vi "Verify Blink HE.vi"(0 "GEA2 Reference In":refnum<k24>, 1 "SSD":string, 2 "Blinking LED":T1, 5 "Initial Timeout (s)":dbl, 7 "Retry Count":i32, 9 "Max Blink Rate (sec)":dbl, 11 "Error In":errorcluster, 13 "Ignore Brightness?":bool) -> (4 "GEA2 Reference Out":refnum<k24>, 6 "Pass/Fail?":bool, 8 "Report Text":string, 10 "Blink Times (s)":dbl[](array[numeric]), 15 "Error Out":errorcluster)   [LabVIEW 2016, in "TLMB.lvlib"]
doc: "This VI is used to verify that a particular LED is blinking on the HEUI."
uses:
  Projects/TLMB.lvlib
  Q:/Common/DLLs/GEA3/GeaCommunication.dll
  Common/DLLs/GEA3/GeaCommunication.dll
  controls/HEUI_Display_Blink.ctl
  Common/LabVIEW GEA2 Toolkit/LabVIEW_GEA2_Toolkit.lvlibp/type defs/Source_Destination.ctl
  Common/LabVIEW GEA2 Toolkit/LabVIEW_GEA2_Toolkit.lvlibp
panel:
  in  "Standalone":bool
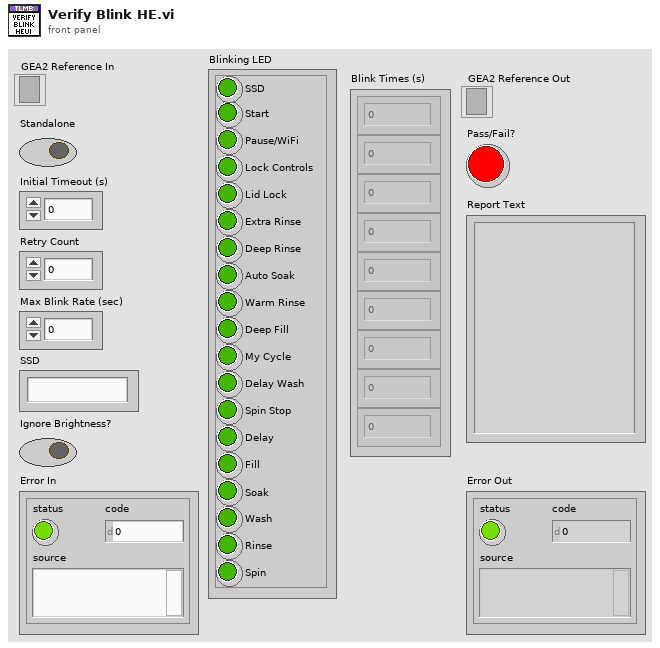
[diagram p1: front panel]
types:
  T1 = typedef "TLMB.lvlib/HEUI_Display_Blink.ctl" = cluster{"Start":bool, "Pause/WiFi":bool, "Lock Controls":bool, "Lid Lock":bool, "Extra Rinse":bool, "Deep Rinse":bool, "Auto Soak":bool, "Warm Rinse":bool, "Deep Fill":bool, "My Cycle":bool, "Delay Wash":bool, "Spin Stop":bool, "Delay":bool, "Fill":bool, "Soak":bool, "Wash":bool, "Rinse":bool, "Spin":bool, "SSD":bool}
  T2 = typedef "LabVIEW_GEA2_Toolkit.lvlibp/Source_Destination.ctl" = cluster{"Source":u8, "Destination":u8}
  T3 = typedef "TLMB.lvlib/HEUI_Display_Care.ctl" = cluster{"SSD":bool, "Cycle Selection":bool, "Stain Selection":bool, "Temp Level":bool, "Soil Level":bool, "Spin Level":bool, "750 Status":bool, "Start":bool, "Pause/WiFi":bool, "Lock Controls":bool, "Lid Lock":bool, "Extra Rinse":bool, "Deep Rinse":bool, "Auto Soak":bool, "Warm Rinse":bool, "Deep Fill":bool, "My Cycle":bool, "Delay Wash":bool, "Spin Stop":bool, "Delay":bool, "Fill":bool, "Soak":bool, "Wash":bool, "Rinse":bool, "Spin":bool}
  T4 = typedef "TLMB.lvlib/HEUI_Display.ctl" = cluster{"SSD":string, "Cycle Selection":T5, "Stain Selection":T6, "Temp Level":T7, "Soil Level":T8, "Spin Level":T9, "750 Status":T10, "Start":bool, "Pause/WiFi":bool, "Lock Controls":bool, "Lid Lock":bool, "Extra Rinse":bool, "Deep Rinse":bool, "Auto Soak":bool, "Warm Rinse":bool, "Deep Fill":bool, "My Cycle":bool, "Delay Wash":bool, "Spin Stop":bool, "Delay":bool, "Fill":bool, "Soak":bool, "Wash":bool, "Rinse":bool, "Spin":bool}
  T5 = typedef "TLMB.lvlib/Cycle Selection Enum.ctl" = enum16{"Colors", "Easy Care", "Delicates", "Hand Wash", "Active Wear", "Speed Wash", "Rinse and Spin", "Drain and Spin", "Basket Clean", "Jeans", "Heavy Duty", "Bulky Items", "Towels", "Whites", "Off", "*Incorrect*"}
  T6 = typedef "TLMB.lvlib/Stain Enum.ctl" = enum16{"Tomato", "Wine", "Blood", "Grass", "Dirt", "Off", "*Incorrect*"}
  T7 = typedef "TLMB.lvlib/Temp Enum.ctl" = enum16{"Hot", "Warm", "Colors", "Cool", "Cold", "Tap Cold", "Off", "*Incorrect*"}
  T8 = typedef "TLMB.lvlib/Soil Enum.ctl" = enum16{"Extra Heavy", "Heavy", "Normal", "Light", "Off", "*Incorrect*"}
  T9 = typedef "TLMB.lvlib/Spin Enum.ctl" = enum16{"Max Spin", "More Spin", "Normal Spin", "No Spin", "Off", "*Incorrect*"}
  T10 = typedef "TLMB.lvlib/750 Status Enum.ctl" = enum16{"Fill", "Wash", "Rinse", "Spin", "Off", "*Incorrect*"}
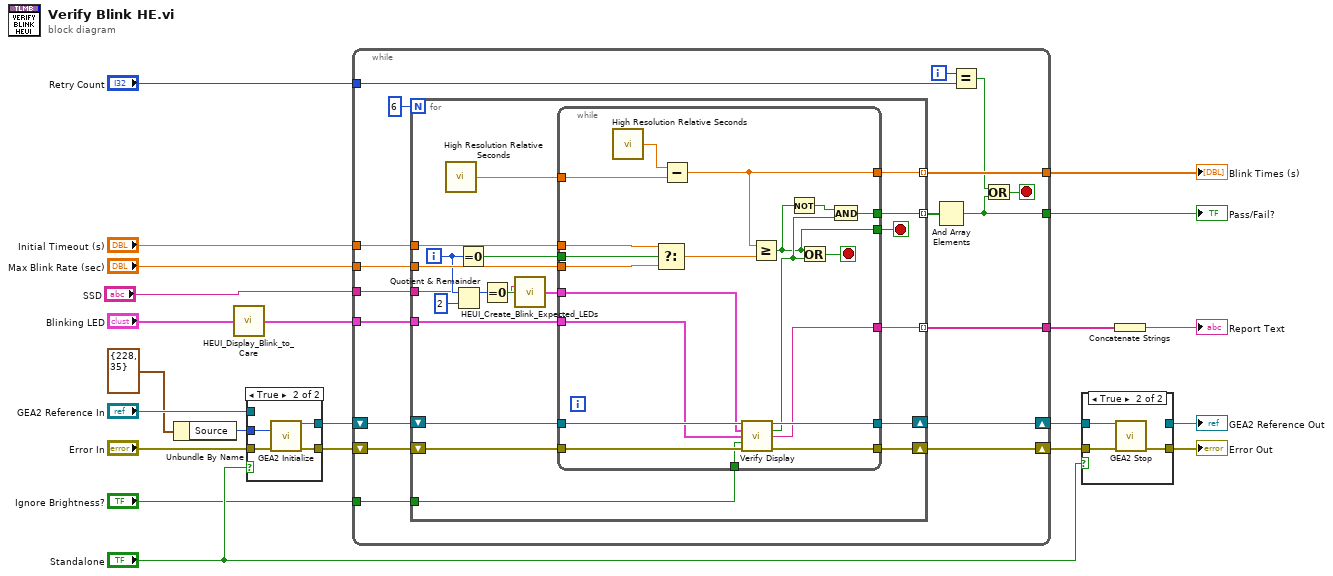
[diagram p0: block diagram]
diagram:
  n1 = Unbundle By Name(T2 {"Source"=228, "Destination"=35} ("GEA Inputs")) -> ("Source"=w21:u8)
  n2 = call "HEUI_Display_Blink_to_Care.vi"("HEUI_Display_Blink"="Blinking LED") -> ("Care?"=w3:T3)  [unwired: 14 in]
  n3 = case shown="True" "Standalone" {
    tunnel: "Error In" -> [w24 w28]
    tunnel: w21 -> [_ w27]
    tunnel: [w23 w26] -> w13
    tunnel: [w24 w25] -> w12
    tunnel: "GEA2 Reference In" -> [w23 _]
    frame False {
    }
    frame True {
      n4 = call "GEA2 Initialize.vi"("Source Address"=w27, "error in"=w28) -> ("GEA2 Reference Out"=w26:refnum<k24>, "error out"=w25:errorcluster)  [unwired: 11 in, 1 out]
    }
  }
  n5 = while {
    tunnel: "Max Blink Rate (sec)" -> [w46]
    tunnel: [w35] -> w7
    tunnel: [w45] -> w14
    tunnel: w3 -> [w40]
    tunnel: "Initial Timeout (s)" -> [w39]
    shift-right: [w42] -> w11
    shift-left: w13 -> [w44]
    shift-right: [w41] -> w10
    shift-left: w12 -> [w43]
    tunnel: [w38] -> w8
    tunnel: "Retry Count" -> [w32]
    tunnel: "Ignore Brightness?" -> [w31]
    tunnel: "SSD" -> [w29]
    i -> [w33]
    stop <- w34 stop-if-true
    n6 = for {
      N: 6 -> [_]
      shift-right: [w65] -> w41
      shift-left: w43 -> [w66]
      shift-right: [w64] -> w42
      shift-left: w44 -> [w63]
      tunnel: w46 -> [w61]
      tunnel: [w59] -> w37 mode=indexing
      tunnel: [w55] -> w38 mode=indexing
      tunnel: [w60] -> w45 mode=indexing
      tunnel: w40 -> [w54]
      tunnel: w39 -> [w57]
      tunnel: w31 -> [w56]
      tunnel: w29 -> [w47]
      i -> [w48]
      stop <- w49 stop-if-true
      n7 = call <vilib>:"High Resolution Relative Seconds.vi"() -> ("relative seconds"=w62:dbl)
      n8 = Quotient & Remainder(x=w48, y=2) -> (x-y*floor(x/y)=w52:i32)  [unwired: 1 out]
      n9 = Equal To 0?(x=w48) -> (x = 0?=w58:bool)
      n10 = Equal To 0?(x=w52) -> (x = 0?=w51:bool)
      n11 = call "HEUI_Create_Blink_Expected_LEDs.vi"("SSD"=w47, "Boolean"=w51) -> ("Expected LEDs Out"=w50:T4)  [unwired: 13 in]
      n12 = while {
        tunnel: w66 -> [w74]
        tunnel: [w73] -> w65
        tunnel: [w75] -> w64
        tunnel: w63 -> [w76]
        tunnel: w62 -> [w85]
        tunnel: w61 -> [w80]
        tunnel: [w83] -> w59
        tunnel: [w84] -> w60
        tunnel: w58 -> [w77]
        tunnel: w54 -> [w72]
        tunnel: w57 -> [w81]
        tunnel: w56 -> [w70]
        tunnel: [w69] -> w55
        tunnel: w50 -> [w71]
        tunnel: [w67] -> w49
        stop <- w82 stop-if-true
        n13 = call <vilib>:"High Resolution Relative Seconds.vi"() -> ("relative seconds"=w86:dbl)
        n14 = Select(t=w81, s=w77, f=w80) -> (s? t:f=w79:dbl)
        n15 = Subtract(x=w86, y=w85) -> (x-y=w84:dbl)
        n16 = call "Verify Display.vi"("GEA2 Reference In"=w76, "Expected LEDs"=w71, "Care?"=w72, "Ignore Brightness?"=w70, "Error In"=w74) -> ("GEA2 Reference Out"=w75:refnum<k24>, "Pass/Fail?"=w68:bool, "Report Text"=w69:string, "Error Out"=w73:errorcluster)  [unwired: 7 in]
        n17 = Greater Or Equal?(x=w84, y=w79) -> (x >= y?=w67:bool)
        n18 = Not(x=w67) -> (.not. x?=w78:bool)
        n19 = Or(x=w67, y=w68) -> (x .or. y?=w82:bool)
        n20 = And(x=w78, y=w68) -> (x .and. y?=w83:bool)
      }
    }
    n21 = And Array Elements(Boolean array=w37) -> (logical AND=w35:bool)
    n22 = Equal?(x=w33, y=w32) -> (x = y?=w36:bool)
    n23 = Or(x=w36, y=w35) -> (x .or. y?=w34:bool)
  }
  "Pass/Fail?" <- w7
  "Blink Times (s)" <- w14
  n24 = case shown="True" "Standalone" {
    tunnel: w10 -> [w88 w91]
    tunnel: [w88 w90] -> w19
    tunnel: w11 -> [w87 w89]
    tunnel: [w87 _] -> w17
    frame False {
    }
    frame True {
      n25 = call "GEA2 Stop.vi"("GEA2 Reference In"=w89, "Error In"=w91) -> ("Error Out"=w90:errorcluster)  [unwired: 13 in]
    }
  }
  "GEA2 Reference Out" <- w17
  "Error Out" <- w19
  n26 = Concatenate Strings(w8) -> (→"Report Text":string)
